vi "_test_ValidateSchema.vi"(10 "XML schema path":path=path "C:/Users/Administrator/Desktop/GIT/Ballard-Arinc-429-XML-Generator/Source/Assemblies/Ballard_Parameter_ni/ARINC429_Parameters_XML_Schema.xsd", 11 "XML path":path) -> (0 "error out":errorcluster, 3 "ValidateAgainstXMLSchema":bool)   [LabVIEW 2020]
uses:
  C:/Users/Administrator/Desktop/GIT/Ballard-Arinc-429-XML-Generator/Source/Assemblies/Ballard_Parameter_ni/bin/Debug/Parameters_Arinc429_XML_Tools.dll
  Source/Assemblies/Ballard_Parameter_ni/bin/Debug/Parameters_Arinc429_XML_Tools.dll
  <vilib>/addons/_JKI Toolkits/Caraya/classes/Assert/Assert True.vi
  <vilib>/addons/_JKI Toolkits/Caraya/classes/Test/Test.lvclass
  <vilib>/addons/_JKI Toolkits/Caraya/classes/Assert/Assert.lvclass
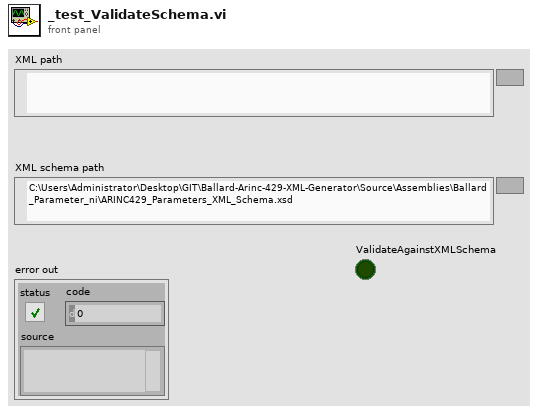
[diagram p1: front panel]
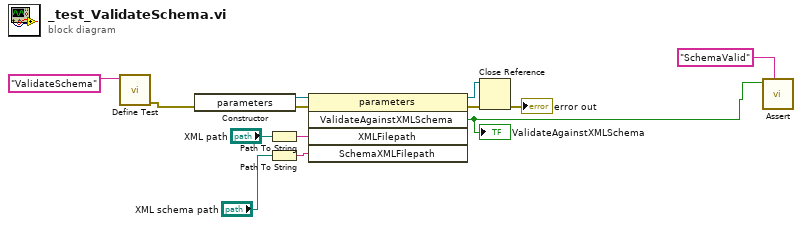
[diagram p0: block diagram]
diagram:
  n1 = call <vilib>:"Define Test.vi"("Label (VI Title)"="ValidateSchema") -> ("error out"=w3:errorcluster)  [unwired: 10 in]
  n2 = constructor class="parameters"(error in=w3) -> (reference out=w13:refnum<k24>, error out=w6:errorcluster)  [unwired: 2 in, 1 out]
  n3 = Path To String(path="XML path") -> (string=w10:string)
  n4 = Path To String(path="XML schema path") -> (string=w9:string)
  n5 = invoke class="parameters" method="ValidateAgainstXMLSchema"(reference=w13, error in=w6, "XMLFilepath"=w10, "SchemaXMLFilepath"=w9) -> (reference out=w8:refnum<k24>, error out=w7:errorcluster, "ValidateAgainstXMLSchema"=w2:bool)  [unwired: 1 in, 2 out]
  "ValidateAgainstXMLSchema" <- w2
  n6 = Close Reference(reference=w8, error in (no error)=w7) -> (error out=→"error out":errorcluster)
  n7 = call-poly <vilib>:"Assert.vi"("Label"="SchemaValid", "True?"=w2) -> ()  [unwired: 9 in, 1 out]
